vi "navX Open.vi"(5 "I2C Bus":T6=enum."I2C MXP", 7 "SPI Bus":T4=enum."SPI MXP", 8 "error in":errorcluster, 10 "Update Rate (4Hz-60Hz)":T15=50 min=4 max=60 step=1, 11 "navX Interface Protocol":T2) -> (0 "error out":errorcluster, 1 "Opened?":bool, 3 "navX Device TypeDef":T1={"navX Interface Protocol"=enum."SPI", "navX Interface Protocol TypeDefs"={"SPIDevRef"={"DevStatus"={"status"=FALSE, "code"=0, "source"=""}, "Handle"=0, "SPI Bus"=enum."SPI On-Board, CS0"}, "I2CDevRef"={"DevStatus"={"status"=FALSE, "code"=0, "source"=""}, "Device Address"=0, "Handle"=0, "I2C Bus"=enum."Invalid"}}, "navX System Information"={"Board Information"={"WhoAmI (50 | 0x32)"=0, "Board Revision"=0, "Firmware Major Version"=0, "Firmware Minor Version"=0, "NAVX_BOARD_CAPABILITY"={"OMNIMOUNT"=FALSE, "YAW_RESET"=FALSE, "VEL_AND_DISP"=FALSE}, "NAVX_BOARD_YAW_AXIS"={"BOARD_YAW_AXIS_UP"=FALSE, "BOARD_YAW_AXIS"=0}}, "Status"={"Update Rate Hz"=0, "Accelerometer Full-Scale Range"=0, "Gyro Full-Scale Range"=0, "NAVX_OP_STATUS"=0, "NAVX_CAL_STATUS"=0, "NAVX_SELFTEST_STATUS"=0, "NAVX_SENSOR_STATUS"={"MOVING"=FALSE, "YAW_STABLE"=FALSE, "MAG_DISTURBANCE"=FALSE, "ALTITUDE_VALID"=FALSE, "SEALEVEL_PRESS_SET"=FALSE, "FUSED_HEADING_VALID"=FALSE}}, "Offsets"={"Yaw"=0.0, "Quat W"=0.0, "Quat X"=0.0, "Quat Y"=0.0, "Quat Z"=0.0}, "LastSampleTimestamp"=0.0, "LastSampleValid"=FALSE}, "navX Common Information"={"Update Rate (4Hz-60Hz)"=50, "refnum name"="", "error"={"status"=FALSE, "code"=0, "source"=""}, "LastSampleFPGATimestamp"=0.0}} {"navX Common Information"."Update Rate (4Hz-60Hz)" min=4 max=60 step=1; "navX System Information"."Status"."NAVX_OP_STATUS" items=["INITIALIZING", "SELFTEST_IN_PROGRESS", "ERROR", "IMU_AUTOCAL_IN_PROGRESS", "NORMAL"]; "navX System Information"."Status"."NAVX_CAL_STATUS" items=["IMU_CAL_STATE_MASK"=3, "IMU_CAL_INPROGRESS"=0, "IMU_CAL_ACCUMULATE"=1, "IMU_CAL_COMPLETE"=2, "MAG_CAL_COMPLETE"=4, "BARO_CAL_COMPLETE"=8]; "navX Interface Protocol TypeDefs"."I2CDevRef"."Device Address" format="%.0x"})   [LabVIEW 2015, in "navX-MXP IMU.lvlib"]
doc: "This VI is used to open the connection to a navX MXP unit over SPI or I2C."
uses:
  navX-MXP IMU.lvlib
  TypeDefs/Value TypeDefs/navX Interface Protocol.ctl
  TypeDefs/Value TypeDefs/navX Update Rate.ctl
  <vilib>/Rock Robotics/SystemInterfaces/spilib/spi_bus.ctl
  <vilib>/Rock Robotics/SystemInterfaces/i2clib/i2c_bus.ctl
  TypeDefs/navX Device TypeDef.ctl
  <vilib>/Rock Robotics/WPI/SPI/WPI_SPIDevRef.ctl
  <vilib>/Rock Robotics/WPI/I2C/WPI_I2CDevRef.ctl
  TypeDefs/Data TypeDefs/navX Board Information.ctl
  TypeDefs/Value TypeDefs/navX NAVX_BOARD_CAPABILITY.ctl
  TypeDefs/Value TypeDefs/navX NAVX_BOARD_YAW_AXIS.ctl
  TypeDefs/Data TypeDefs/navX Status Data.ctl
  TypeDefs/Value TypeDefs/navX NAVX_OP_STATUS.ctl
  TypeDefs/Value TypeDefs/navX NAVX_CAL_STATUS.ctl
  TypeDefs/Value TypeDefs/navX NAVX_SENSOR_STATUS.ctl
  TypeDefs/Data TypeDefs/navX Offsets Data.ctl
  <vilib>/Rock Robotics/SystemInterfaces/NetworkCommunication/NetComm_UsageReport_ResourceType.ctl
  TypeDefs/Value TypeDefs/navX Device Registers.ctl
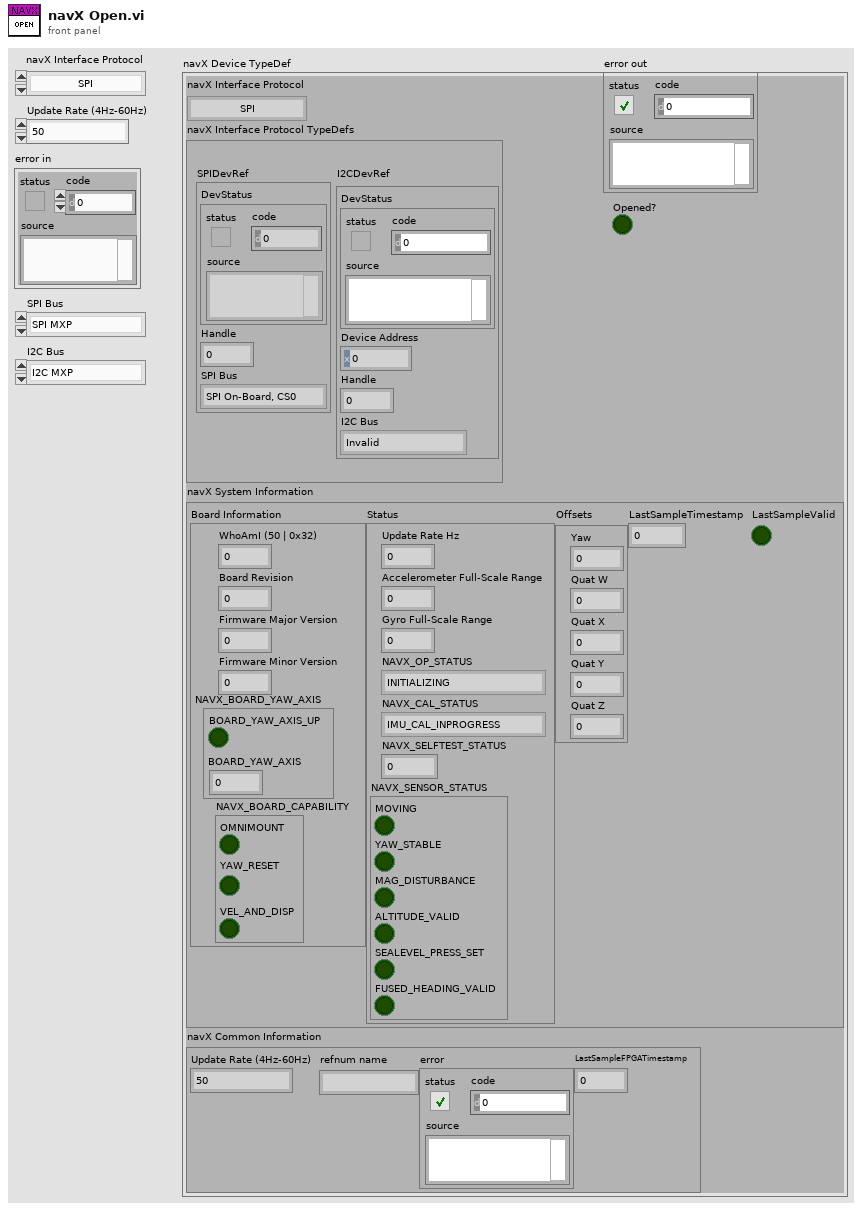
[diagram p1: front panel]
types:
  T1 = typedef "navX-MXP IMU.lvlib/navX Device TypeDef.ctl" = cluster{"navX Interface Protocol":T2, "navX Interface Protocol TypeDefs":cluster{"SPIDevRef":T3, "I2CDevRef":T5}, "navX System Information":cluster{"Board Information":T7, "Status":T10, "Offsets":T14, "LastSampleTimestamp":dbl, "LastSampleValid":bool}, "navX Common Information":cluster{"Update Rate (4Hz-60Hz)":T15, "refnum name":string, "error":errorcluster, "LastSampleFPGATimestamp":dbl}}
  T2 = typedef "navX-MXP IMU.lvlib/navX Interface Protocol.ctl" = enum16{"SPI", "I2C", "SERIAL"}
  T3 = typedef "WPI_SPIDevRef.ctl" = cluster{"DevStatus":errorcluster, "Handle":i32, "SPI Bus":T4}
  T4 = typedef "spi_bus.ctl" = enum16{"SPI On-Board, CS0", "SPI On-Board, CS1", "SPI On-Board, CS2", "SPI On-Board, CS3", "SPI MXP", "Invalid"}
  T5 = typedef "WPI_I2CDevRef.ctl" = cluster{"DevStatus":errorcluster, "Device Address":u8, "Handle":i32, "I2C Bus":T6}
  T6 = typedef "i2c_bus.ctl" = enum16{"I2C On-Board", "I2C MXP", "Invalid"}
  T7 = typedef "navX-MXP IMU.lvlib/navX Board Information.ctl" = cluster{"WhoAmI (50 | 0x32)":u8, "Board Revision":u8, "Firmware Major Version":u8, "Firmware Minor Version":u8, "NAVX_BOARD_CAPABILITY":T8, "NAVX_BOARD_YAW_AXIS":T9}
  T8 = typedef "navX-MXP IMU.lvlib/navX NAVX_BOARD_CAPABILITY.ctl" = cluster{"OMNIMOUNT":bool, "YAW_RESET":bool, "VEL_AND_DISP":bool}
  T9 = typedef "navX-MXP IMU.lvlib/navX NAVX_BOARD_YAW_AXIS.ctl" = cluster{"BOARD_YAW_AXIS_UP":bool, "BOARD_YAW_AXIS":u8}
  T10 = typedef "navX-MXP IMU.lvlib/navX Status Data.ctl" = cluster{"Update Rate Hz":u8, "Accelerometer Full-Scale Range":u8, "Gyro Full-Scale Range":u16, "NAVX_OP_STATUS":T11, "NAVX_CAL_STATUS":T12, "NAVX_SELFTEST_STATUS":u8, "NAVX_SENSOR_STATUS":T13}
  T11 = typedef "navX-MXP IMU.lvlib/navX NAVX_OP_STATUS.ctl" = u8
  T12 = typedef "navX-MXP IMU.lvlib/navX NAVX_CAL_STATUS.ctl" = u8
  T13 = typedef "navX-MXP IMU.lvlib/navX NAVX_SENSOR_STATUS.ctl" = cluster{"MOVING":bool, "YAW_STABLE":bool, "MAG_DISTURBANCE":bool, "ALTITUDE_VALID":bool, "SEALEVEL_PRESS_SET":bool, "FUSED_HEADING_VALID":bool}
  T14 = typedef "navX-MXP IMU.lvlib/navX Offsets Data.ctl" = cluster{"Yaw":dbl, "Quat W":dbl, "Quat X":dbl, "Quat Y":dbl, "Quat Z":dbl}
  T15 = typedef "navX-MXP IMU.lvlib/navX Update Rate.ctl" = u8
  T16 = typedef "NetComm_UsageReport_ResourceType.ctl" = enum8{"Controller", "Module", "Language", "CANPlugin", "Accelerometer", "ADXL345", "AnalogChannel", "AnalogTrigger", "AnalogTriggerOutput", "CANJaguar", "Compressor", "Counter", "Dashboard", "DigitalInput", "DigitalOutput", "DriverStationCIO", "DriverStationEIO", "DriverStationLCD", "Encoder", "GearTooth", "Gyro", "I2C", "Framework", "Jaguar", "Joystick", "Kinect", "KinectStick", "PIDController", "Preferences", "PWM", "Relay", "RobotDrive", "SerialPort", "Servo", "Solenoid", "SPI", "Task", "Ultrasonic", "Victor", "Button", "Command", "AxisCamera", "PCVideoServer", "SmartDashboard", "Talon", "HiTechnicColorSensor", "HiTechnicAccel", "HiTechnicCompass", "SRF08", "AnalogOutput", "Victor SP", "Talon SRX", "CAN Talon SRX"}
  T17 = typedef "navX-MXP IMU.lvlib/navX Device Registers.ctl" = u8
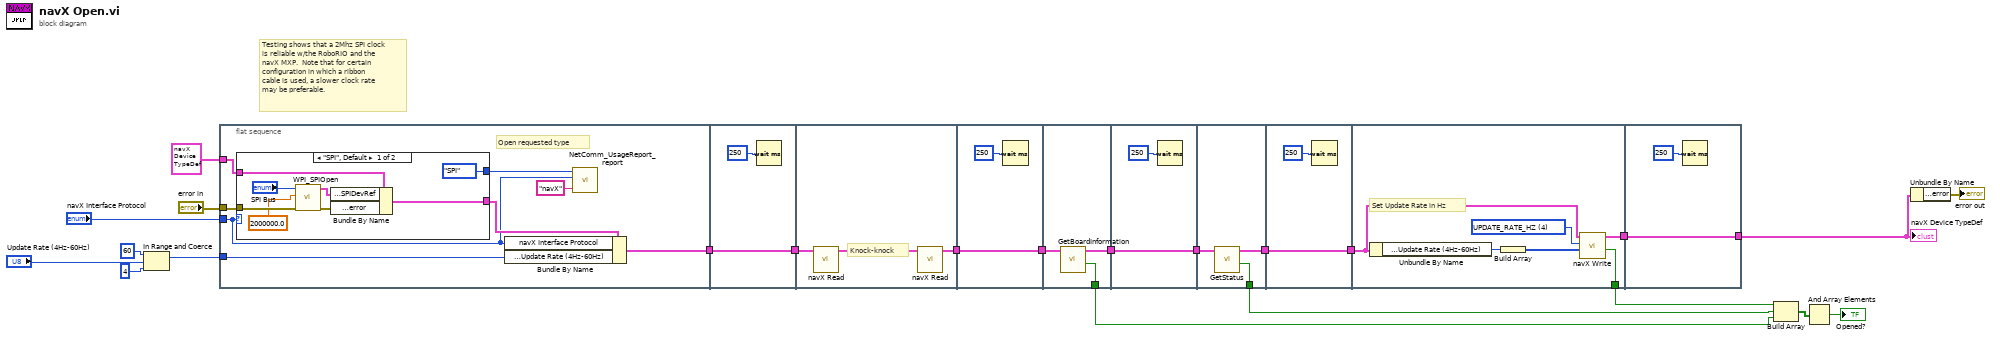
[diagram p0: block diagram]
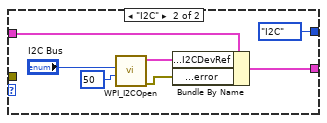
[diagram p2: hidden frame]
diagram:
  # "Testing shows that a 2Mhz SPI clock is reliable w/the RoboRIO and the navX MXP.  Note that for certain configuration in which a ribbon cable is used, a slower clock rate may be preferable."
  n1 = In Range and Coerce(upper limit=u8 60, x="Update Rate (4Hz-60Hz)", lower limit=u8 4) -> (coerced(x)=w11:T15)  [unwired: 1 out]
  n2 = flat-sequence {
    tunnel: "navX Interface Protocol" -> [w25]
    tunnel: T1 {"navX Interface Protocol"=enum."SPI", "navX Interface Protocol TypeDefs"={"SPIDevRef"={"DevStatus"={"status"=FALSE, "code"=0, "source"=""}, "Handle"=0, "SPI Bus"=enum."SPI On-Board, CS0"}, "I2CDevRef"={"DevStatus"={"status"=FALSE, "code"=0, "source"=""}, "Device Address"=0, "Handle"=0, "I2C Bus"=enum."Invalid"}}, "navX System Information"={"Board Information"={"WhoAmI (50 | 0x32)"=0, "Board Revision"=0, "Firmware Major Version"=0, "Firmware Minor Version"=0, "NAVX_BOARD_CAPABILITY"={"OMNIMOUNT"=FALSE, "YAW_RESET"=FALSE, "VEL_AND_DISP"=FALSE}, "NAVX_BOARD_YAW_AXIS"={"BOARD_YAW_AXIS_UP"=FALSE, "BOARD_YAW_AXIS"=0}}, "Status"={"Update Rate Hz"=0, "Accelerometer Full-Scale Range"=0, "Gyro Full-Scale Range"=0, "NAVX_OP_STATUS"=0, "NAVX_CAL_STATUS"=0, "NAVX_SELFTEST_STATUS"=0, "NAVX_SENSOR_STATUS"={"MOVING"=FALSE, "YAW_STABLE"=FALSE, "MAG_DISTURBANCE"=FALSE, "ALTITUDE_VALID"=FALSE, "SEALEVEL_PRESS_SET"=FALSE, "FUSED_HEADING_VALID"=FALSE}}, "Offsets"={"Yaw"=0.0, "Quat W"=0.0, "Quat X"=0.0, "Quat Y"=0.0, "Quat Z"=0.0}, "LastSampleTimestamp"=0.0, "LastSampleValid"=FALSE}, "navX Common Information"={"Update Rate (4Hz-60Hz)"=50, "refnum name"="", "error"={"status"=FALSE, "code"=0, "source"=""}, "LastSampleFPGATimestamp"=0.0}} ("navX Device TypeDef") -> [w31]
    tunnel: "error in" -> [w29]
    tunnel: w11 -> [w27]
    tunnel: [w28] -> w16
    tunnel: w16 -> [w48]
    tunnel: [w48] -> w15
    tunnel: w15 -> [w51]
    tunnel: [w49] -> w17
    tunnel: w17 -> [w52]
    tunnel: [w52] -> w18
    tunnel: w18 -> [w55]
    tunnel: [w56] -> w6
    tunnel: [w54] -> w1
    tunnel: w6 -> [w58]
    tunnel: [w58] -> w5
    tunnel: w5 -> [w60]
    tunnel: [w61] -> w7
    tunnel: [w59] -> w2
    tunnel: w7 -> [w62]
    tunnel: [w62] -> w3
    tunnel: [w65] -> w8
    tunnel: [w66] -> w4
    tunnel: w3 -> [w64]
    tunnel: [w71] -> w20
    tunnel: w4 -> [w71]
    frame #0 {
      # "Open requested type"
      n3 = case shown="\"SPI\", Default" w25 {
        tunnel: w31 -> [w39 w46]
        tunnel: [w36 w45] -> w30
        tunnel: w29 -> [w35 _]
        tunnel: [NetComm_UsageReport_ResourceType."SPI" ("Resource Type") NetComm_UsageReport_ResourceType."I2C" ("Resource Type")] -> w26
        frame "SPI", Default {
          n4 = call <vilib>:"WPI_SPIOpen.vi"("error in"=w35, "Clock Rate (Hz)"=2000000.0, "SPI Bus"="SPI Bus") -> ("error out"=w38:errorcluster, "SPIDevRef"=w37:T3)  [unwired: 7 in]
          n5 = Bundle By Name(cluster=w39, "navX Interface Protocol TypeDefs.SPIDevRef"=w37, "navX Common Information.error"=w38) -> (w36:T1)
        }
        frame "I2C" {
          n6 = call <vilib>:"WPI_I2COpen.vi"("Device Address"=u8 50, "I2C Bus"="I2C Bus") -> ("error out"=w44:errorcluster, "I2CDevRef"=w43:T5)  [unwired: 8 in]
          n7 = Bundle By Name(cluster=w46, "navX Interface Protocol TypeDefs.I2CDevRef"=w43, "navX Common Information.error"=w44) -> (w45:T1)
        }
      }
      n8 = Bundle By Name(cluster=w30, "navX Interface Protocol"=w25, "navX Common Information.Update Rate (4Hz-60Hz)"=w27) -> (w28:T1)
      n9 = call <vilib>:"NetComm_UsageReport_report.vi"("Feature"="navX", "Instance Number"=w25, "Resource Type"=w26) -> ()  [unwired: 9 in]
    }
    frame #1 {
      n10 = Wait (ms)(milliseconds to wait=u32 250) -> ()  [unwired: 1 out]
    }
    frame #2 {
      # "Knock-knock"
      n11 = call "navX Read.vi"("navX Device TypeDef"=w51) -> ("navX Device TypeDef"=w50:T1)  [unwired: 8 in, 2 out]
      n12 = call "navX Read.vi"("navX Device TypeDef"=w50) -> ("navX Device TypeDef"=w49:T1)  [unwired: 8 in, 2 out]
    }
    frame #3 {
      n13 = Wait (ms)(milliseconds to wait=u32 250) -> ()  [unwired: 1 out]
    }
    frame #4 {
      n14 = call "GetBoardInformation.vi"("navX Device TypeDef"=w55) -> ("Valid?"=w54:bool, "navX Device TypeDef"=w56:T1)  [unwired: 8 in, 1 out]
    }
    frame #5 {
      n15 = Wait (ms)(milliseconds to wait=u32 250) -> ()  [unwired: 1 out]
    }
    frame #6 {
      n16 = call "GetStatus.vi"("navX Device TypeDef"=w60) -> ("Valid?"=w59:bool, "navX Device TypeDef"=w61:T1)  [unwired: 8 in, 1 out]
    }
    frame #7 {
      n17 = Wait (ms)(milliseconds to wait=u32 250) -> ()  [unwired: 1 out]
    }
    frame #8 {
      w69 = T17 4 items=["WHOAMI"=0, "HW_REV"=1, "FW_VER_MAJOR"=2, "FW_VER_MINOR"=3, "UPDATE_RATE_HZ"=4, "ACCEL_FSR_G"=5, "GYRO_FSR_DPS"=6, "OP_STATUS"=8, "CAL_STATUS"=9, "SELFTEST_STATUS"=10, "SENSOR_STATUS"=16, "TIMESTAMP"=18, "YAW"=22, "PITCH"=24, "ROLL"=26, "HEADING"=28, "FUSED_HEADING"=30, "ALTITUDE_I"=32, "ALTITUDE_D"=34, "LINERA_ACC_X"=36, "LINERA_ACC_Y"=38, "LINERA_ACC_Z"=40, "QUAT_W"=42, "QUAT_X"=44, "QUAT_Y"=46, "QUAT_Z"=48, "MPU_TEMP_C"=50, "GYRO_X"=52, "GYRO_Y"=54, "GYRO_Z"=56, "ACC_X"=58, "ACC_Y"=60, "ACC_Z"=62, "MAG_X"=64, "MAG_Y"=66, "MAG_Z"=68, "PRESSURE_I"=70, "PRESSURE_D"=72, "PRESSURE_TEMP"=74, "YAW_OFFSET"=76, "QUAT_OFFSET_W"=78, "QUAT_OFFSET_X"=80, "QUAT_OFFSET_Y"=82, "QUAT_OFFSET_Z"=84] ("Device Register")
      # "Set Update Rate in Hz"
      n18 = Unbundle By Name(w64) -> ("navX Common Information.Update Rate (4Hz-60Hz)"=w68:T15)
      n19 = Build Array(w68) -> (w67:T15[])
      n20 = call "navX Write.vi"("navX Message"=w67, "Device Register"=w69, "navX Device TypeDef"=w64) -> ("Valid?"=w65:bool, "navX Device TypeDef"=w66:T1)  [unwired: 7 in]
    }
    frame #9 {
      n21 = Wait (ms)(milliseconds to wait=u32 250) -> ()  [unwired: 1 out]
    }
  }
  n22 = Build Array(w8, w2, w1) -> (w10:bool[])
  n23 = And Array Elements(Boolean array=w10) -> (logical AND=→"Opened?":bool)
  n24 = Unbundle By Name(w20) -> ("navX Common Information.error"=→"error out":errorcluster)
  "navX Device TypeDef" <- w20
